vi "Create GB 2014-11-20.vi"(5 "Max # of atoms":i32=9999999, 6 "Edge Duplication Range":dbl=3.0, 7 "Skip cleanup if no subset":bool=TRUE, 8 "Reduce to Repeating":T2={"Slab X"=4.6, "Slab Y"=4.0, "Tolerance (A)"=0.5, "Presorted?"=FALSE}, 9 "Min Seperation Distance (A)":dbl=2.0, 10 "Grain Growth and Geometry":T3={"Grain 1 Length (A)"=6.0, "Grain 2 Length (A)"=6.0, "Max Grain Height (A)"=90.0, "Max Grain Width (A)"=90.0, "Grain 1 Start"=-0.001, "Overlap Region (A)"=0.001}, 11 "Grain Boundary Definition":T4={"Grain 1 Orientation"=[1.0, 0.6019417241891012, 0.029651947654046266], "Grain 2 Orientation"=[1.0, 0.730727623275494, 0.2205637301176], "Twist Angle (Deg)"=0.0, "Translation Vector"=[0.0, 0.0, 0.0]}) -> (0 "GB Data":string[][](array[string])=[["Grain 1, h", "Grain 1, k", "Grain 1, L", "Grain 2, h", "Grain 2, k", "Grain 2, L", "Twist Angle (Deg)", "Translation Tx", "Translation Ty", "Translation Tz", "Tilt Angle (Deg)", "Viewing Angle, h", "Viewing Angle, k", "Viewing Angle, L", "Grain 1 Length (factor)", "Grain 2 Length (factor", "Max Grain Height (A)", "Max Grain Width (A)", "Grain 1 Start", "Overlap Region (A)", "Reduction Slab X", "Reduction Slab Y", "Reduction Tolerance (A)", "Min Atomic Separation Distance", "Edge Duplication Range", "# Atoms"], ["1.000000", "0.601942", "0.029652", "1.000000", "0.730728", "0.220564", "0.000000", "0.000000", "0.000000", "0.000000", "10.024930", "1.000000", "-1.661290", "0.000000", "1.000000", "1.000000", "90.000000", "90.000000", "-0.001000", "0.001000", "4.600000", "4.000000", "0.500000", "2.000000", "3.000000", "12135.000000"]], 1 "Reduced Orthorhombic?":bool, 2 "Reduced Rhombahedral?":bool, 3 "Grain Boundary":T5={"Structure Name"="(0.00) twist [1.000,0.602,0.030] [1.000,0.731,0.221] (0.00,0.00,0.00)T GB", "Lattice vector a"=[270.03, 0.0, 0.0], "Lattice vector b"=[0.0, 270.03, 0.0], "Lattice vector c"=[0.0, 0.0, 6.006], "Atoms Array"=[{"Atom Name"="Cd", "Positions (Direct)"=array6055x3[18165 elements], "Positions (Cartesian)"=array6055x3[18165 elements]}, {"Atom Name"="Te", "Positions (Direct)"=array6080x3[18240 elements], "Positions (Cartesian)"=array6080x3[18240 elements]}], "# of atoms"=12135} {"Atoms Array"."Positions (Cartesian)" format="%#_4f"; "Atoms Array"."Positions (Direct)" format="%#_4f"}, 4 "Creation Time":T1={"Time to create primitives"=0, "Time to Grow to Box"=4152, "Time to find subset"=1109, "Time to Cleanup"=1})   [LabVIEW 2010]
uses:
  <vilib>/Analysis/NI_AALPro.lvlib
  <vilib>/Analysis/_algsub.llb/Real Vector Norm.vi
  <vilib>/Analysis/NI_AALBase.lvlib
  <vilib>/Analysis/baseanly.llb/Real A x B.vi
  <vilib>/Analysis/baseanly.llb/A x Vector.vi
panel:
  out "error out":errorcluster
  out "Original # of atoms":i32=12135
  in  "Expansion Factor":dbl=1.0
  out "Expected # of Atoms":i32=166
  in  "Integer Tolerance":dbl=0.01
  in  "Predict Best Size":bool
  in  "Headers":string[](array[string])=["Grain 1, h", "Grain 1, k", "Grain 1, L", "Grain 2, h", "Grain 2, k", "Grain 2, L", "Twist Angle (Deg)", "Translation Tx", "Translation Ty", "Translation Tz", "Tilt Angle (Deg)", "Viewing Angle, h", "Viewing Angle, k", "Viewing Angle, L", "Grain 1 Length (factor)", "Grain 2 Length (factor", "Max Grain Height (A)", "Max Grain Width (A)", "Grain 1 Start", "Overlap Region (A)", "Reduction Slab X", "Reduction Slab Y", "Reduction Tolerance (A)", "Min Atomic Separation Distance", "Edge Duplication Range", "# Atoms"]
  out "Rhombehedral Atoms":i32=12135
  out "Orthorhombic atoms":i32=12135
  out "Time to Cleanup":u32=1
  out "Time to find subset":u32=1109
  out "Time to Grow to Box":u32=4152
  out "Time to create primitives":u32
  out "Tilt Angle":dbl=10.024929742348679
  out "# of Atoms Removed":i32=28
  out "Repeating Y Length Scale":dbl=13.227303403298492
  out "Repeating X Length Scale":dbl
  out "Mutual Viewing Angle":dbl[](array[numeric])=[1.0, -1.6612903871170226, 0.0]
  in  "Conventional Unit Cell":T5={"Structure Name"="CdTe", "Lattice vector a"=[6.615785553057252, 0.0, 0.0], "Lattice vector b"=[0.0, 6.615785553057252, 0.0], "Lattice vector c"=[0.0, 0.0, 6.615785553057252], "Atoms Array"=[{"Atom Name"="Cd", "Positions (Direct)"=[[0.0, 0.0, 0.0], [0.0, 0.5, 0.5], [0.5, 0.0, 0.5], [0.5, 0.5, 0.0]], "Positions (Cartesian)"=[[0.0, 0.0, 0.0], [0.0, 3.307892776528626, 3.307892776528626], [3.307892776528626, 0.0, 3.307892776528626], [3.307892776528626, 3.307892776528626, 0.0]]}, {"Atom Name"="Te", "Positions (Direct)"=[[0.25, 0.25, 0.25], [0.75, 0.75, 0.25], [0.75, 0.25, 0.75], [0.25, 0.75, 0.75]], "Positions (Cartesian)"=[[1.653946388264313, 1.653946388264313, 1.653946388264313], [4.96183916479294, 4.96183916479294, 1.653946388264313], [4.96183916479294, 1.653946388264313, 4.96183916479294], [1.653946388264313, 4.96183916479294, 4.96183916479294]]}], "# of atoms"=8}
  # "Primitives"
  # "Grain Growth"
  # "Make into repeating cell"
  # "Remove Collisions"
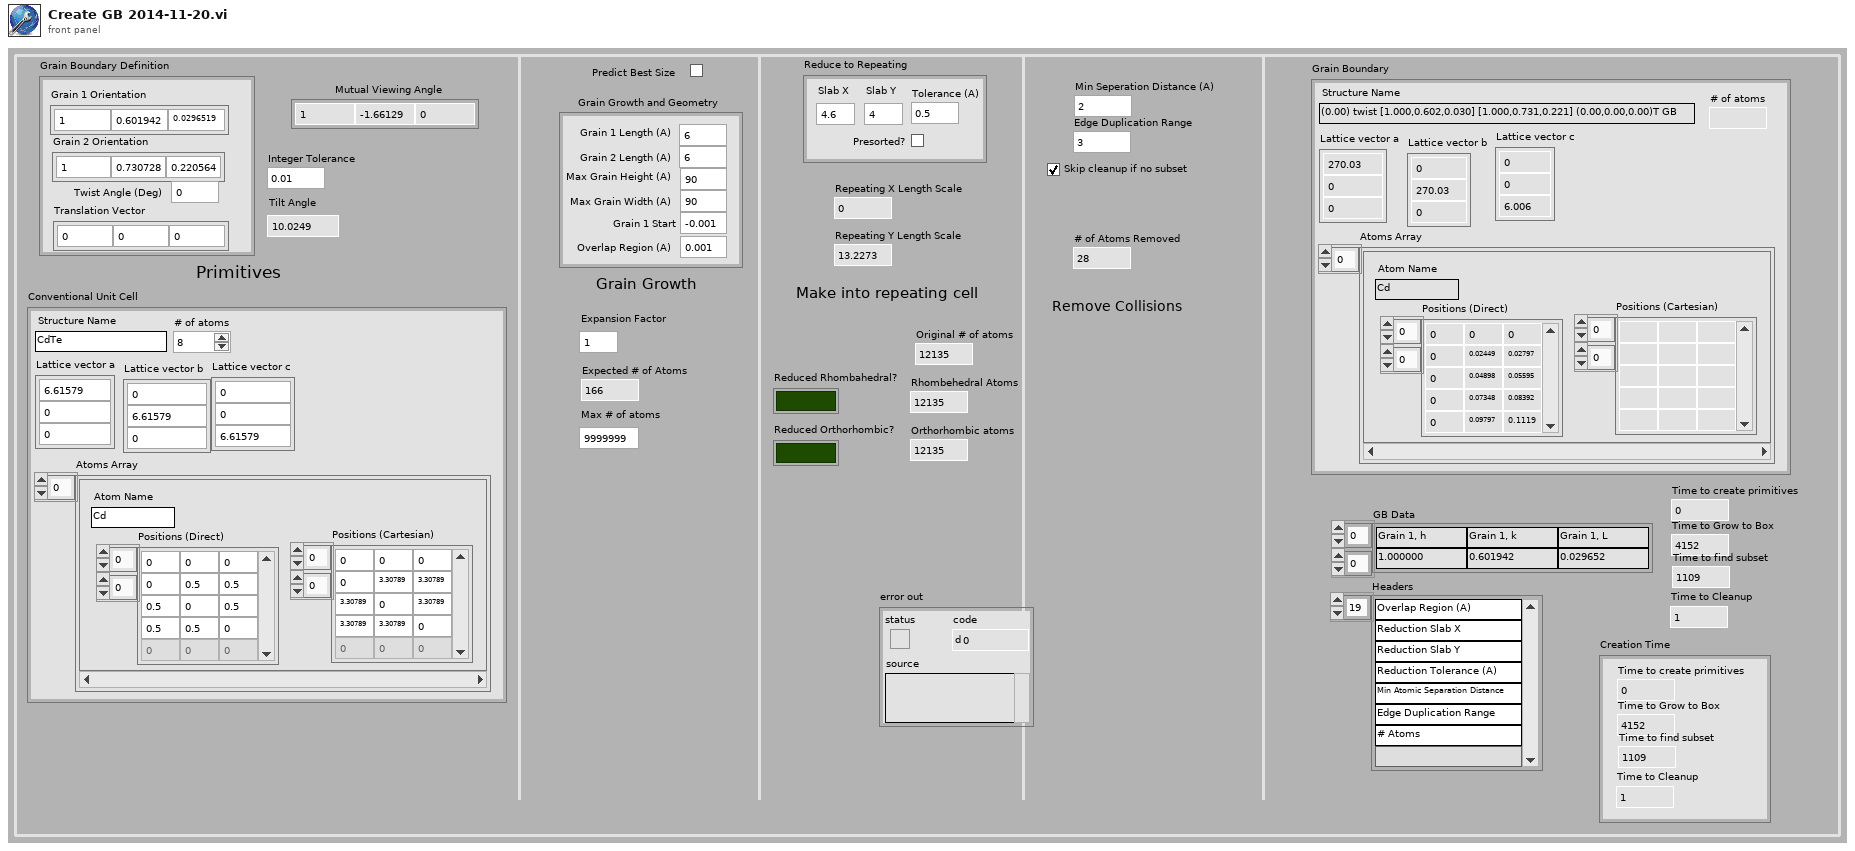
[diagram p1: front panel]
types:
  T1 = cluster{"Time to create primitives":u32, "Time to Grow to Box":u32, "Time to find subset":u32, "Time to Cleanup":u32}
  T2 = cluster{"Slab X":dbl, "Slab Y":dbl, "Tolerance (A)":dbl, "Presorted?":bool}
  T3 = cluster{"Grain 1 Length (A)":dbl, "Grain 2 Length (A)":dbl, "Max Grain Height (A)":dbl, "Max Grain Width (A)":dbl, "Grain 1 Start":dbl, "Overlap Region (A)":dbl}
  T4 = cluster{"Grain 1 Orientation":dbl[], "Grain 2 Orientation":dbl[], "Twist Angle (Deg)":dbl, "Translation Vector":dbl[]}
  T5 = cluster{"Structure Name":string, "Lattice vector a":dbl[], "Lattice vector b":dbl[], "Lattice vector c":dbl[], "Atoms Array":cluster{"Atom Name":string, "Positions (Direct)":dbl[][], "Positions (Cartesian)":dbl[][]}[], "# of atoms":i32}
  T6 = cluster{"Grain 1 Orientation":dbl[], "Grain 2 Orientation":dbl[], "Twist Angle (Deg)":dbl}
  T7 = typedef "NI_Matrix.lvlib/RealMatrix.ctl" = dbl[][]
  T8 = cluster{"Z Min":dbl, "Max Grain Width (A)":dbl, "Z Min":dbl, "Max Grain Height (A)":dbl, "Grain 1 Start":dbl, "# of Atoms":i32}
  T9 = cluster{"Z Min":dbl, "Max Grain Width (A)":dbl, "Z Min":dbl, "Max Grain Height (A)":dbl, dbl, void}
  T10 = cluster{"Z Min":dbl, void, "Z Min":dbl, void, "Grain 1 Start":dbl, void}
  T11 = cluster{"Z Min":dbl, void, "Z Min":dbl, void, "Grain 1 Start":dbl, "# of Atoms":i32}
  T12 = cluster{"Z Min":dbl, "Max Grain Width (A)":dbl, "Z Min":dbl, "Max Grain Height (A)":dbl, "Grain 1 Start":dbl, "# of Atoms":dbl}
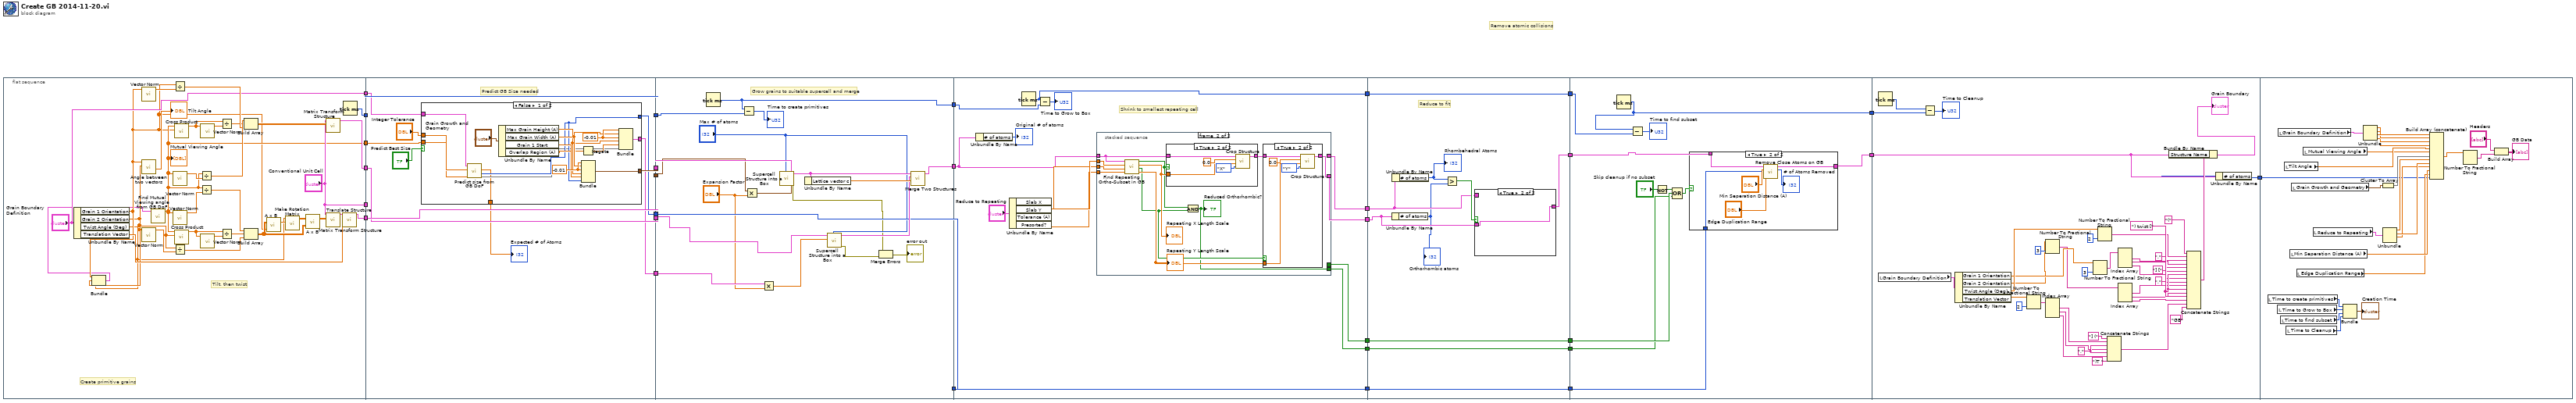
[diagram p0: block diagram]
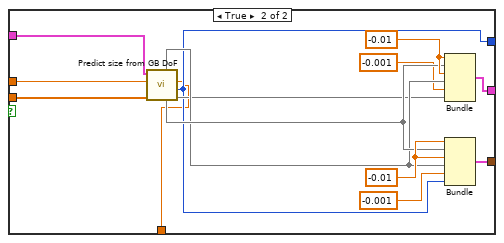
[diagram p2: hidden frame]
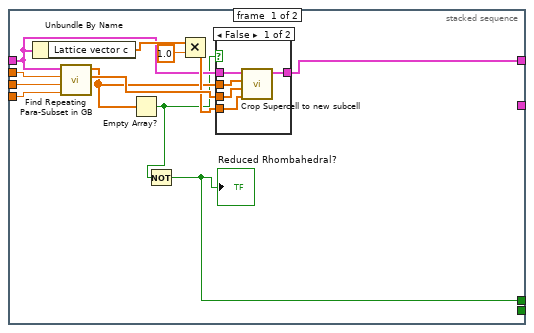
[diagram p3: hidden frame]
diagram:
  # "Remove atomic collisions"
  n1 = flat-sequence {
    tunnel: [w42] -> w12
    tunnel: [w53] -> w11
    tunnel: [w39] -> w10
    tunnel: ["Conventional Unit Cell"] -> w9
    tunnel: [w35] -> w8
    tunnel: ["Grain Boundary Definition"] -> w7
    tunnel: w12 -> [w72]
    tunnel: [w72] -> w6
    tunnel: w11 -> [w71]
    tunnel: [w71] -> w5
    tunnel: w10 -> [w70]
    tunnel: [w70] -> w4
    tunnel: w9 -> [_]
    tunnel: w8 -> [w69]
    tunnel: w7 -> [w68]
    tunnel: [w66] -> w3
    tunnel: [w65] -> w2
    tunnel: [w64] -> w1
    tunnel: w6 -> [w120]
    tunnel: w5 -> [w121]
    tunnel: [w116] -> w28
    tunnel: w4 -> [w114]
    tunnel: [w113] -> w27
    tunnel: [w112] -> w25
    tunnel: w3 -> [w111]
    tunnel: w2 -> [w109]
    tunnel: w1 -> [w112]
    tunnel: w28 -> [w125]
    tunnel: [w127] -> w24
    tunnel: w27 -> [w134]
    tunnel: [w132] -> w22
    tunnel: w25 -> [w131]
    tunnel: [w131] -> w20
    tunnel: [w126] -> w18
    tunnel: [w124] -> w16
    tunnel: [w123] -> w15
    tunnel: w24 -> [w183]
    tunnel: [w181] -> w23
    tunnel: w22 -> [w186]
    tunnel: [w186] -> w21
    tunnel: w20 -> [w185]
    tunnel: [w185] -> w19
    tunnel: w18 -> [w182]
    tunnel: w16 -> [w177]
    tunnel: w15 -> [w178]
    tunnel: [w178] -> w14
    tunnel: [w177] -> w13
    tunnel: w23 -> [w199]
    tunnel: [w198] -> w29
    tunnel: w21 -> [w196]
    tunnel: [w195] -> w26
    tunnel: w19 -> [w193]
    tunnel: w14 -> [w190]
    tunnel: w13 -> [w189]
    tunnel: w29 -> [w217]
    tunnel: w26 -> [w218]
    tunnel: [w216] -> w17
    tunnel: w17 -> [w257]
    frame #0 {
      # "Tilt, then twist"
      # "Create primitive grains"
      n2 = Unbundle By Name("Grain Boundary Definition") -> ("Grain 1 Orientation"=w33:dbl[], "Grain 2 Orientation"=w32:dbl[], "Twist Angle (Deg)"=w31:dbl, "Translation Vector"=w40:dbl[])
      n3 = Bundle("Grain 1 Orientation"=w33, "Grain 2 Orientation"=w32, "Twist Angle (Deg)"=w31) -> (w30:T6)  [unwired: 1 in]
      n4 = call-poly <vilib>:"Vector Norm.vi"("Input Vector"=w33) -> ("norm"=w59:dbl)  [unwired: 9 in, 1 out]
      n5 = call "Angle between two vectors.vi"("Vector 2"=w32, "Vector 1"=w33) -> ("Angle (Degrees)"=→"Tilt Angle":dbl)  [unwired: 7 in, 2 out]
      n6 = call-poly <vilib>:"Vector Norm.vi"("Input Vector"=w32) -> ("norm"=w45:dbl)  [unwired: 9 in, 1 out]
      n7 = call "Find Mutual Viewing angle from GB DoF.vi"("Grain Boundary Macro DoF"=w30) -> ("Mutual Viewing Angle"=w35:dbl[])  [unwired: 8 in, 2 out]
      "Mutual Viewing Angle" <- w35
      n8 = Divide(x=w33, y=w59) -> (x/y=w57:dbl[])
      n9 = call-poly <vilib>:"Vector Norm.vi"("Input Vector"=w35) -> ("norm"=w61:dbl)  [unwired: 9 in, 1 out]
      n10 = call-poly <vilib>:"Vector Norm.vi"("Input Vector"=w35) -> ("norm"=w43:dbl)  [unwired: 9 in, 1 out]
      n11 = Divide(x=w32, y=w45) -> (x/y=w47:dbl[])
      n12 = call <vilib>:"Cross Product.vi"("B Vector"=w33, "A Vector"=w35) -> ("Cross Product"=w55:dbl[])  [unwired: 8 in, 1 out]
      n13 = call <vilib>:"Cross Product.vi"("B Vector"=w32, "A Vector"=w35) -> ("Cross Product"=w48:dbl[])  [unwired: 8 in, 1 out]
      n14 = Divide(x=w35, y=w61) -> (x/y=w58:dbl[])
      n15 = Divide(x=w35, y=w43) -> (x/y=w46:dbl[])
      n16 = call-poly <vilib>:"Vector Norm.vi"("Input Vector"=w55) -> ("norm"=w60:dbl)  [unwired: 9 in, 1 out]
      n17 = call-poly <vilib>:"Vector Norm.vi"("Input Vector"=w48) -> ("norm"=w44:dbl)  [unwired: 9 in, 1 out]
      n18 = Divide(x=w55, y=w60) -> (x/y=w54:dbl[])
      n19 = Divide(x=w48, y=w44) -> (x/y=w52:dbl[])
      n20 = Build Array(w58, w54, w57) -> (w56:T7)
      n21 = Build Array(w46, w52, w47) -> (w37:T7)
      n22 = call-poly <vilib>:"A x B.vi"("Vector"=w33, "A"=w37) -> ("A x Vector"=w36:dbl[])  [unwired: 1 out]
      n23 = call "Make Rotation Matrix.vi"("Rotation Axis"=w36, "Rotation Angle (Degree)"=w31) -> ("Rotation Matrix"=w50:T7)  [unwired: 9 in]
      n24 = call-poly <vilib>:"A x B.vi"("B"=w37, "A"=w50) -> ("A x B"=w49:T7)  [unwired: 1 out]
      n25 = call "Matrix Transform Structure.vi"("Matrix Transform"=w56, "Original Structure"="Conventional Unit Cell") -> ("After Transform"=w53:T5)  [unwired: 9 in]
      n26 = call "Matrix Transform Structure.vi"("Matrix Transform"=w49, "Original Structure"="Conventional Unit Cell") -> ("After Transform"=w51:T5)  [unwired: 9 in]
      n27 = call "Translate Structure.vi"("Translation Vector (Cartesian)"=w40, "Atomic Structure"=w51) -> ("Shifted Structure"=w42:T5)  [unwired: 9 in]
      n28 = Tick Count (ms)() -> (millisecond timer value=w39:u32)
    }
    frame #1 {
      # "Predict GB Size needed"
      n29 = case shown="False" "Predict Best Size" {
        tunnel: w69 -> [w76 w102]
        tunnel: w68 -> [w77 w101]
        tunnel: [w85 w98] -> w66
        tunnel: [w79 w92] -> w65
        tunnel: [w75 w91] -> w64
        tunnel: "Integer Tolerance" -> [w78 w90]
        tunnel: [w73 w89] -> w62
        frame False {
          w84 = -0.01 ("Z Min")
          w87 = -0.01 ("Z Min")
          n30 = call "Predict size from GB DoF.vi"("Integer Tolerance"=w76, "Mutual Viewing Angle"=w78, "Grain Boundary Definition"=w77) -> (0:w74, "# of Atoms"=w75:i32, "Expected Volume (A3)"=w73:dbl)  [unwired: 5 in, 1 out]
          n31 = Unbundle By Name("Grain Growth and Geometry") -> ("Max Grain Height (A)"=w82:dbl, "Max Grain Width (A)"=w83:dbl, "Grain 1 Start"=w86:dbl, "Overlap Region (A)"=w81:dbl)
          n32 = Negate(x=w81) -> (-x=w80:dbl)
          n33 = Bundle("Z Min"=w87, "Max Grain Width (A)"=w83, "Z Min"=w87, "Max Grain Height (A)"=w82, "Grain 1 Start"=w86, "# of Atoms"=w75) -> (w85:T8)  [unwired: 1 in]
          n34 = Bundle("Z Min"=w84, "Max Grain Width (A)"=w83, "Z Min"=w84, "Max Grain Height (A)"=w82, w80, w74) -> (w79:T9)  [unwired: 1 in]
        }
        frame True {
          w97 = -0.01 ("Z Min")
          w100 = -0.01 ("Z Min")
          n35 = call "Predict size from GB DoF.vi"("Integer Tolerance"=w102, "Mutual Viewing Angle"=w90, "Grain Boundary Definition"=w101) -> (0:w93, "# of Atoms"=w91:i32, "Expected Volume (A3)"=w89:dbl, 4:w96, 5:w95)  [unwired: 3 in, 1 out]
          n36 = Bundle("Z Min"=w97, w96, "Z Min"=w97, w95, "Grain 1 Start"=-0.001, w93) -> (w92:T10)  [unwired: 1 in]
          n37 = Bundle("Z Min"=w100, w96, "Z Min"=w100, w95, "Grain 1 Start"=-0.001, "# of Atoms"=w91) -> (w98:T11)  [unwired: 1 in]
        }
      }
      "Expected # of Atoms" <- w62
    }
    frame #2 {
      # "Grow grains to suitable supercell and merge"
      n38 = Tick Count (ms)() -> (millisecond timer value=w113:u32)
      n39 = Subtract(x=w113, y=w114) -> (x-y=→"Time to create primitives":u32)
      n40 = Multiply(x=w111, y="Expansion Factor") -> (x*y=w110:T12)
      n41 = Multiply(x=w109, y="Expansion Factor") -> (x*y=w107:dbl)
      n42 = call "Supercell Structure into a Box.vi"("Max # of atoms"="Max # of atoms", "Draw Box"=w110, "Subcrystal"=w121) -> ("error out"=w105:errorcluster, "Expanded cubic Structure"=w117:T5)  [unwired: 6 in, 1 out]
      n43 = Unbundle By Name(w117) -> ("Lattice vector c"=w119:dbl[])
      n44 = call "Supercell Structure into a Box.vi"("Max # of atoms"="Max # of atoms", "Draw Box"=w107, "Subcrystal"=w120) -> ("error out"=w104:errorcluster, "Expanded cubic Structure"=w118:T5)  [unwired: 6 in, 1 out]
      n45 = Merge Errors(w105, w104) -> (→"error out":errorcluster)
      n46 = call "Merge Two Structures.vi"("Translation Vector (1 to 2)"=w119, "Atomic Structure 2"=w118, "Atomic Structure 1"=w117) -> ("Atomic Structure of 1 + 2 by T"=w116:T5)  [unwired: 8 in]
    }
    frame #3 {
      # "Shrink to smallest repeating cell"
      n47 = Unbundle By Name(w125) -> ("# of atoms"=→"Original # of atoms":i32)
      n48 = Unbundle By Name("Reduce to Repeating") -> ("Slab X"=w130:dbl, "Slab Y"=w129:dbl, "Tolerance (A)"=w128:dbl)  [unwired: 1 out]
      n49 = Tick Count (ms)() -> (millisecond timer value=w132:u32)
      n50 = Subtract(x=w132, y=w134) -> (x-y=→"Time to Grow to Box":u32)
      n51 = stacked-sequence {
        tunnel: [w139 _] -> w127
        tunnel: w130 -> [w142 w164]
        tunnel: w129 -> [w141 w163]
        tunnel: w128 -> [w140 w162]
        tunnel: w125 -> [w143 w161]
        tunnel: [_ w157] -> w126
        tunnel: [_ w154] -> w124
        tunnel: [w136 _] -> w123
        frame #0 {
          n52 = Unbundle By Name(w143) -> ("Lattice vector c"=w145:dbl[])
          n53 = call "Find Repeating Para-Subset in GB.vi"("Tolerance (A)"=w140, "Slab Y"=w141, "Slab X"=w142, "Supercell Structure"=w143) -> ("New Lattice Vector b"=w147:dbl[], "New Lattice Vector a"=w138:dbl[])  [unwired: 5 in, 1 out]
          n54 = Empty Array?(array=w138) -> (empty?=w137:bool)
          n55 = Not(x=w137) -> (.not. x?=w136:bool)
          "Reduced Rhombahedral?" <- w136
          n56 = Multiply(x=w145, y=1.0) -> (x*y=w144:dbl[])
          n57 = case shown="False" w137 {
            tunnel: w147 -> [w152 _]
            tunnel: w138 -> [w151 _]
            tunnel: w144 -> [w150 _]
            tunnel: w143 -> [w149 w153]
            tunnel: [w148 w153] -> w139
            frame False {
              n58 = call "Crop Supercell to new subcell.vi"("New Lattice Vector c"=w150, "New Lattice Vector b"=w152, "New Lattice Vector a"=w151, "Supercell Structure"=w149) -> ("Reduced Structure"=w148:T5)  [unwired: 7 in]
            }
            frame True {
            }
          }
        }
        frame #1 {
          n59 = call "Find Repeating Ortho-Subset in GB.vi"("Tolerance (A)"=w162, "Slab Y"=w163, "Slab X"=w164, "Grain Boundary"=w161) -> ("Repeating Y Length Scale"=w158:dbl, "Subset Y found?!"=w155:bool, "Repeating X Length Scale"=w159:dbl, "Subset X found?!"=w156:bool)  [unwired: 4 in]
          "Repeating X Length Scale" <- w159
          "Repeating Y Length Scale" <- w158
          n60 = case shown="True" w156 {
            tunnel: w161 -> [w171 w176]
            tunnel: [w171 w173] -> w160
            tunnel: w159 -> [_ w172]
            frame False {
            }
            frame True {
              n61 = call "Crop Structure.vi"("Cropping Index"=enum16{"X", "Y", "Z"}."X", "Upper Bound Z"=w172, "Lower bound Z"=0.0, "Input Structure"=w176) -> ("Cropped Structure"=w173:T5)  [unwired: 7 in]
            }
          }
          n62 = And(x=w156, y=w155) -> (x .and. y?=w154:bool)
          "Reduced Orthorhombic?" <- w154
          n63 = case shown="True" w155 {
            tunnel: w160 -> [w165 w170]
            tunnel: w158 -> [_ w168]
            tunnel: [w165 w166] -> w157
            frame False {
            }
            frame True {
              n64 = call "Crop Structure.vi"("Cropping Index"=enum16{"X", "Y", "Z"}."Y", "Upper Bound Z"=w168, "Lower bound Z"=0.0, "Input Structure"=w170) -> ("Cropped Structure"=w166:T5)  [unwired: 7 in]
            }
          }
        }
      }
    }
    frame #4 {
      # "Reduce to fit"
      n65 = Unbundle By Name(w182) -> ("# of atoms"=w179:i32)
      "Orthorhombic atoms" <- w179
      n66 = Unbundle By Name(w183) -> ("# of atoms"=w180:i32)
      "Rhombehedral Atoms" <- w180
      n67 = Greater?(x=w180, y=w179) -> (0:w184:bool)
      n68 = case shown="True" w184 {
        tunnel: [w187 w188] -> w181
        tunnel: w183 -> [w187 _]
        tunnel: w182 -> [_ w188]
        frame False {
        }
        frame True {
        }
      }
    }
    frame #5 {
      n69 = Tick Count (ms)() -> (millisecond timer value=w195:u32)
      n70 = Subtract(x=w195, y=w196) -> (x-y=→"Time to find subset":u32)
      n71 = Not(x="Skip cleanup if no subset") -> (.not. x?=w192:bool)
      n72 = Compound Arithmetic op=OR(w192, w190, w189) -> (w191:bool)
      n73 = case shown="True" w191 {
        tunnel: w199 -> [w200 w204]
        tunnel: [w200 w203] -> w198
        tunnel: w193 -> [_ w201]
        frame False {
        }
        frame True {
          n74 = call "Remove Close Atoms on GB.vi"("Grain Boundary Location (A)"=w201, "Edge Duplication Range"="Edge Duplication Range", "Minimally Allowable Distance (A)"="Min Seperation Distance (A)", "Structure"=w204) -> ("# of Atoms Removed"=→"# of Atoms Removed":i32, "Structure with atoms removed"=w203:T5)  [unwired: 6 in]
        }
      }
    }
    frame #6 {
      w240 = "," ("string")
      w233 = "," ("string")
      n75 = local read "Grain Boundary Definition"() -> (w243:T4)
      n76 = Tick Count (ms)() -> (millisecond timer value=w219:u32)
      n77 = Subtract(x=w219, y=w218) -> (x-y=→"Time to Cleanup":u32)
      n78 = Unbundle By Name(w243) -> ("Grain 1 Orientation"=w213:dbl[], "Grain 2 Orientation"=w210:dbl[], "Twist Angle (Deg)"=w244:dbl, "Translation Vector"=w245:dbl[])
      n79 = Number To Fractional String(number=w245, precision (6)=i16 2) -> (F-format string=w236:string[])  [unwired: 2 in]
      n80 = Number To Fractional String(number=w210, precision (6)=i16 3) -> (F-format string=w209:string[])  [unwired: 2 in]
      n81 = Index Array(array=w236) -> (element #1=w237:string, element #2=w239:string, element #3=w241:string)  [unwired: 3 in]
      n82 = Number To Fractional String(number=w213, precision (6)=i16 3) -> (F-format string=w212:string[])  [unwired: 2 in]
      n83 = Number To Fractional String(number=w244, precision (6)=i16 2) -> (F-format string=w224:string)  [unwired: 2 in]
      n84 = Concatenate Strings("] (" ("string"), w237, w240, w239, w240, w241, ")T " ("string")) -> (w208:string)
      n85 = Index Array(array=w212) -> (element #1=w226:string, element #2=w228:string, element #3=w229:string)  [unwired: 3 in]
      n86 = Index Array(array=w209) -> (element #1=w231:string, element #2=w232:string, element #3=w234:string)  [unwired: 3 in]
      n87 = Concatenate Strings("(" ("string"), w224, ") twist [" ("string"), w226, "," ("string"), w228, w233, w229, "] [" ("string"), w231, w233, w232, w233, w234, w208, "GB" ("string")) -> (w221:string)
      n88 = Bundle By Name(cluster=w217, "Structure Name"=w221) -> (→"Grain Boundary":T5)
      n89 = Unbundle By Name(w217) -> ("# of atoms"=w216:i32)
    }
    frame #7 {
      n90 = local read "Time to create primitives"() -> (w249:u32)
      n91 = local read "Time to Grow to Box"() -> (w248:u32)
      n92 = local read "Grain Boundary Definition"() -> (w270:T4)
      n93 = local read "Time to find subset"() -> (w247:u32)
      n94 = local read "Tilt Angle"() -> (w253:dbl)
      n95 = local read "Time to Cleanup"() -> (w250:u32)
      n96 = local read "Min Seperation Distance (A)"() -> (w259:dbl)
      n97 = local read "Grain Growth and Geometry"() -> (w265:T3)
      n98 = local read "Edge Duplication Range"() -> (w258:dbl)
      n99 = local read "Mutual Viewing Angle"() -> (w252:dbl[])
      n100 = local read "Reduce to Repeating"() -> (w263:T2)
      n101 = Bundle("Time to create primitives"=w249, "Time to Grow to Box"=w248, "Time to find subset"=w247, "Time to Cleanup"=w250) -> (→"Creation Time":T1)  [unwired: 1 in]
      n102 = Unbundle(w270) -> ("Grain 1 Orientation"=w269:dbl[], "Grain 2 Orientation"=w268:dbl[], "Twist Angle (Deg)"=w267:dbl, "Translation Vector"=w266:dbl[])
      n103 = Cluster To Array(cluster=w265) -> (array=w264:dbl[])
      n104 = Unbundle(w263) -> ("Slab X"=w262:dbl, "Slab Y"=w261:dbl, "Tolerance (A)"=w260:dbl)  [unwired: 1 out]
      n105 = Build Array (concatenate)(w269, w268, w267, w266, w253, w252, w264, w262, w261, w260, w259, w258, w257) -> (w256:dbl[])
      n106 = Number To Fractional String(number=w256) -> (F-format string=w255:string[])  [unwired: 3 in]
      n107 = Build Array("Headers", w255) -> (→"GB Data":string[][])
    }
  }
